vi "Add Repo Structure Page.vi"(8 "error in (no error)":errorcluster {"code" format="Error %.0f"}, 11 "VIDoc Printer - Confluence In":refnum<class "VIDoc Printer - Confluence.lvclass">) -> (0 "error out":errorcluster {"code" format="Error %.0f"}, 3 "VIDoc Printer - Confluence Out":refnum<class "VIDoc Printer - Confluence.lvclass">)   [LabVIEW 2023, in "VIDoc Printer - Confluence.lvlib" / "VIDoc Printer - Confluence.lvclass"]
uses:
  VIDoc Printer - Confluence.lvclass
  Confluence Formatting/Types/Format Combo Box.ctl
  VIDoc Printer - Confluence.lvclass/VIDoc Printer - Confluence.ctl
  Confluence Formatting/Confluence Formatting.lvlib
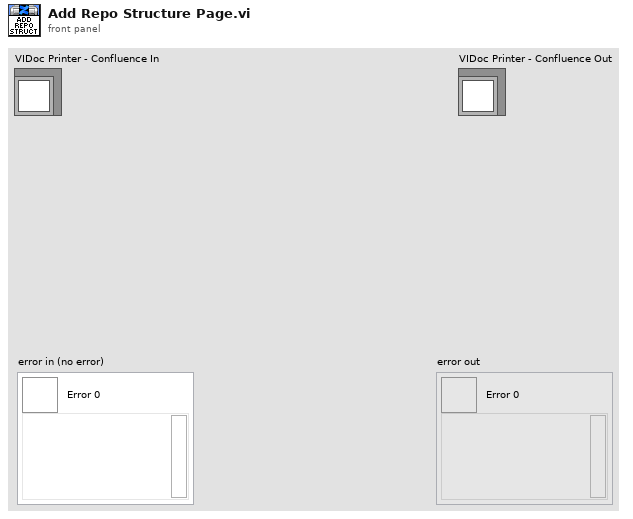
[diagram p1: front panel]
types:
  T1 = typedef "Confluence Formatting.lvlib/Format Combo Box.ctl" = string
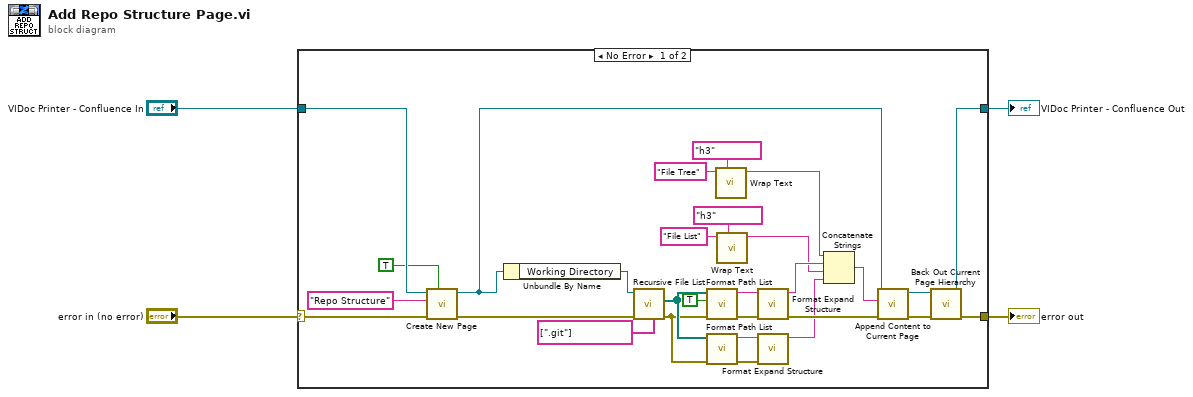
[diagram p0: block diagram]
diagram:
  n1 = case shown="No Error" "error in (no error)" {
    selector: "error in (no error)" -> [w11 w35]
    tunnel: [w30 w35] -> w3
    tunnel: [w17 w34] -> w1
    tunnel: "VIDoc Printer - Confluence In" -> [w9 w34]
    frame No Error {
      n2 = call "Create New Page.vi"("Update Current Page (F)"=TRUE, "error in (no error)"=w11, "Name"="Repo Structure", "VIDoc Printer - Confluence In"=w9) -> ("error out"=w10:errorcluster, "VIDoc Printer - Confluence Out"=w8:refnum<class "VIDoc Printer - Confluence.lvclass">)  [unwired: 4 in, 2 out]
      n3 = Unbundle By Name(w8) -> ("Working Directory"=w29:path)
      n4 = call <vilib>:"Recursive File List.vi"("Folders to Exclude"=string[] [".git"], "error in (no error)"=w10, "Folder Path"=w29) -> ("error out"=w23:errorcluster, "All Files in Dir"=w24:path[])  [unwired: 4 in, 3 out]
      n5 = call "Format Path List.vi"("Error in"=w23, "Tree (F)"=TRUE, "Paths"=w24) -> ("Error out"=w32:errorcluster, "Bullet List String"=w31:string)  [unwired: 7 in]
      n6 = call "Format Path List.vi"("Error in"=w23, "Paths"=w24) -> ("Error out"=w25:errorcluster, "Bullet List String"=w26:string)  [unwired: 8 in]
      n7 = call "Wrap Text.vi"("Formatting"=T1 "h3", "String"="File Tree") -> ("Wrapped String"=w16:string)  [unwired: 8 in, 1 out]
      n8 = call "Wrap Text.vi"("Formatting"=T1 "h3", "String"="File List") -> ("Wrapped String"=w14:string)  [unwired: 8 in, 1 out]
      n9 = call "Format Expand Structure.vi"("Error in"=w32, "Content"=w31) -> ("Error out"=w20:errorcluster, "Expand String"=w15:string)  [unwired: 8 in]
      n10 = call "Format Expand Structure.vi"("Error in"=w25, "Content"=w26) -> ("Expand String"=w13:string)  [unwired: 8 in, 1 out]
      n11 = Concatenate Strings(w16, w15, w14, w13) -> (w12:string)
      n12 = call "Append Content to Current Page.vi"("error in (no error)"=w20, "Content"=w12, "VIDoc Printer - Confluence In"=w8) -> ("error out"=w19:errorcluster, "VIDoc Printer - Confluence Out"=w18:refnum<class "VIDoc Printer - Confluence.lvclass">)  [unwired: 7 in]
      n13 = call "Back Out Current Page Hierarchy.vi"("error in (no error)"=w19, "VIDoc Printer - Confluence In"=w18) -> ("error out"=w30:errorcluster, "VIDoc Printer - Confluence Out"=w17:refnum<class "VIDoc Printer - Confluence.lvclass">)  [unwired: 8 in]
    }
    frame Error {
    }
  }
  "error out" <- w3
  "VIDoc Printer - Confluence Out" <- w1
